vi "APS read d input.vi"(0 "Board_ID":i32, 2 "DI_Group":i32, 3 "DI_Data":i32, 4 "字符串":string, 5 "error in (no error)":errorcluster caption="错误输入（无错误）") -> (14 "function return":i32, 17 "DI_Data out":i32, 18 "元素":bool, 19 "error out":errorcluster caption="错误输出")   [LabVIEW 2012, in "APS168.lvlib"]
doc: "I32 FNTYPE APS_read_d_input(I32 Board_ID, I32 DI_Group, I32 *DI_Data);"
uses:
  APS168.lvlib
  APS168.dll
panel:
  out "数字":i32
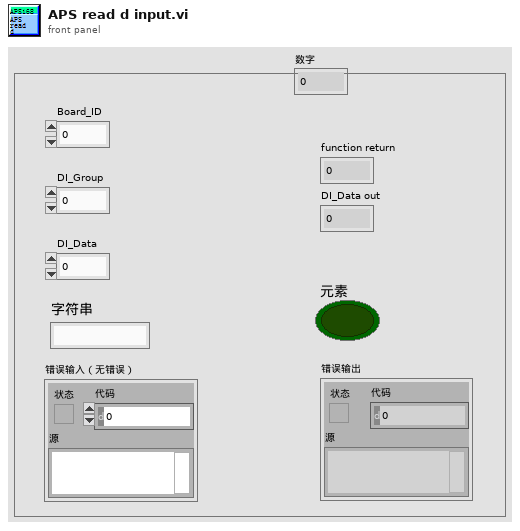
[diagram p1: front panel]
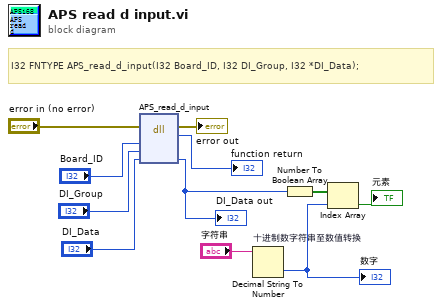
[diagram p0: block diagram]
diagram:
  # "I32 FNTYPE APS_read_d_input(I32 Board_ID, I32 DI_Group, I32 *DI_Data);"
  n1 = dll-call lib="PTH1,abs E\t冲压机运动204c\nAPS168.dll" fn="APS_read_d_input"(error in="error in (no error)", "Board_ID"="Board_ID", "DI_Group"="DI_Group", "DI_Data"="DI_Data") -> (error out=→"error out":errorcluster, "返回类型"=→"function return":i32, "DI_Data"=w1:i32)  [unwired: 4 in, 1 out]
  "DI_Data out" <- w1
  n2 = Decimal String To Number "十进制数字符串至数值转换"(string="字符串") -> (number=w3:i32)  [unwired: 2 in, 1 out]
  "数字" <- w3
  n3 = Number To Boolean Array(number=w1) -> (Boolean array=w5:bool[])
  n4 = Index Array(array=w5, index=w3) -> (element=→"元素":bool)
